vi "Create Long Path.vi"() -> ()   [LabVIEW 2025]
panel:
  out "length":i32
  out "directory copy":path
  out "Array":string[](array[string])
  # "User can browse to and open a VI from a path longer than 255 characters.\n\nUser can successfully load a VI that references a subVI from a path longer than 255 characters.\n\nUser's VI can read and write to a file whose path is longer than 255 characters.\n\nUser's VI can flatten and unflatten a path longer than 255 characters using binary data, JSON, and XML.\n\nUser can build a binary (EXE/DLL/PPL) where source files and output are at paths longer than 255 characters.\n\nUser can build a source distribution where source files and output are at paths longer than 255 characters."
  # "Since at least the Vista timeframe (>10 years ago), \nWindows has supported a “\\\\?\\” path prefix format that allows long paths regardless of the registry key setting. \n\n\n\nLV imposes its own limit before calling the Windows API so we don’t allow leveraging this format. \n\n \n\nWhether you call it a bug or not, it is a behavior we have neglected for over a decade. We could [...] change the file manager to use this prefix internally [...]. This doesn’t impact compatibility so it doesn’t require a breaking release."
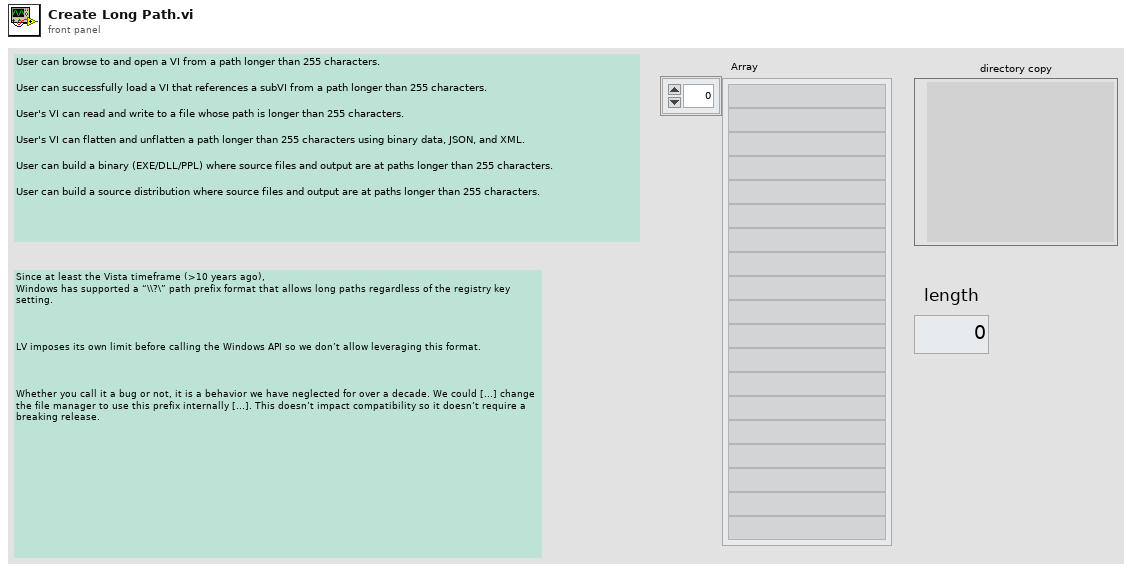
[diagram p1: front panel]
types:
  T1 = enum16{"open", "replace", "create", "open or create", "replace or create", "replace or create with confirmation"}
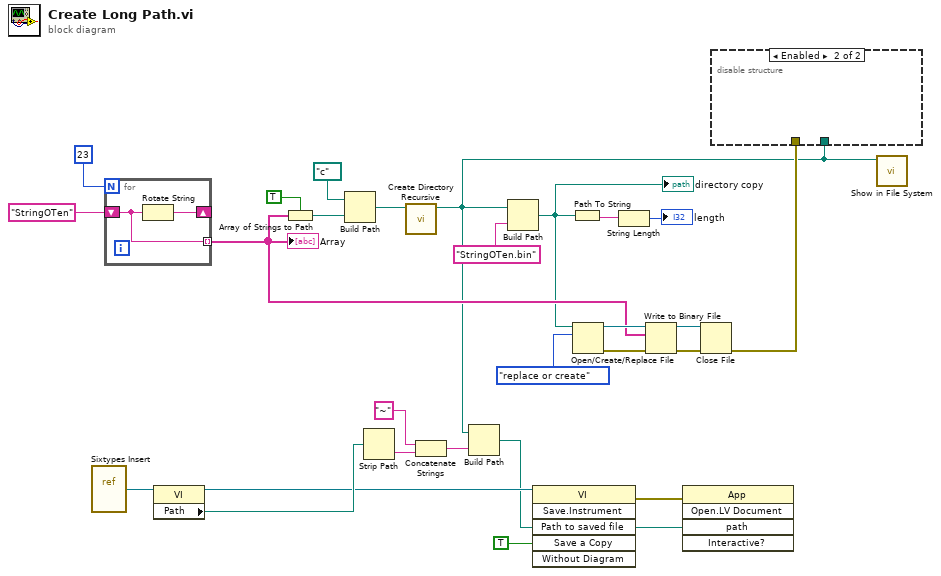
[diagram p0: block diagram]
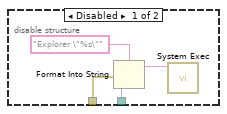
[diagram p2: hidden frame]
diagram:
  n1 = vi-ref "Sixtypes Insert.vi"() -> (w10:refnum<vi>)
  n2 = for {
    N: 23 -> [_]
    tunnel: [w29] -> w18 mode=indexing
    shift-right: [w28] -> _
    shift-left: "StringOTen" -> [w29]
    n3 = Rotate String(1:w29) -> (0:w28:string)
  }
  "Array" <- w18
  n4 = property class="VI"(reference=w10) -> (reference out=w7:refnum<vi>, "Path"=w9:path)  [unwired: 1 in, 1 out]
  n5 = Array of Strings to Path(0:w18, 1:TRUE ("relative")) -> (2:w25:path)
  n6 = Build Path(base path=path "c:/", name or relative path=w25) -> (appended path=w17:path)
  n7 = Strip Path(path=w9) -> (name=w8:string)  [unwired: 1 out]
  n8 = call <vilib>:"Create Directory Recursive.vi"("directory"=w17) -> ("directory copy"=w3:path)  [unwired: 4 in, 2 out]
  n9 = Concatenate Strings("~", w8) -> (w5:string)
  n10 = Build Path(base path=w3, name or relative path=w5) -> (appended path=w2:path)
  n11 = Build Path(base path=w3, name or relative path="StringOTen.bin") -> (appended path=w11:path)
  "directory copy" <- w11
  n12 = invoke class="VI" method="Save.Instrument"(reference=w7, "Path to saved file"=w2, "Save a Copy"=TRUE ("overwrite (F)")) -> (error out=w1:errorcluster)  [unwired: 3 in, 5 out]
  n13 = Path To String(path=w11) -> (string=w13:string)
  n14 = Open/Create/Replace File(file path (use dialog)=w11, operation (0:open)=T1."replace or create") -> (refnum out=w21:refnum<file>, error out=w22:errorcluster)  [unwired: 4 in, 1 out]
  n15 = String Length(string=w13) -> (length=→"length":i32)
  n16 = Write to Binary File(file (use dialog)=w21, data=w18, error in=w22) -> (refnum out=w19:refnum<file>, error out=w20:errorcluster)  [unwired: 3 in, 1 out]
  n17 = invoke class="App" method="Open.LV Document"(error in=w1, "path"=w2) -> ()  [unwired: 3 in, 5 out]
  n18 = Close File(refnum=w19, error in=w20) -> (error out=w14:errorcluster)  [unwired: 1 out]
  n19 = disable-structure shown="Enabled" {
    disable-tunnel: w14 -> [w31 _]
    disable-tunnel: w3 -> [w30 _]
    frame Disabled {
      n20 = Format Into String(format string="Explorer \"%s\"", error in=w31, w30) -> (resulting string=w32:string)  [unwired: 1 in, 1 out]
      n21 = call <vilib>:"System Exec.vi"("command line"=w32) -> ()  [unwired: 7 in, 4 out]
    }
    frame Enabled {
    }
  }
  n22 = call <vilib>:"Show in File System.vi"("file or directory path"=w3) -> ()  [unwired: 10 in, 1 out]
